vi "Line Main.vi"() -> ()   [LabVIEW 2020]
panel:
  in  "Send Image":bool
  in  "Image File Path":path
  out "Reply":string
  in  "Send Message":bool
  in  "Message":string
  in  "Token":string="zqz9UE9y1PFtpszUMYZdfwgDTmGI6nrZ7WZ0uJgGMP1"
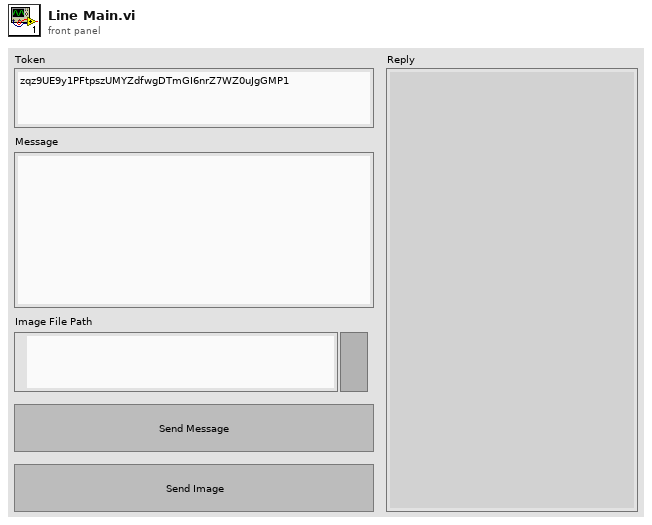
[diagram p1: front panel]
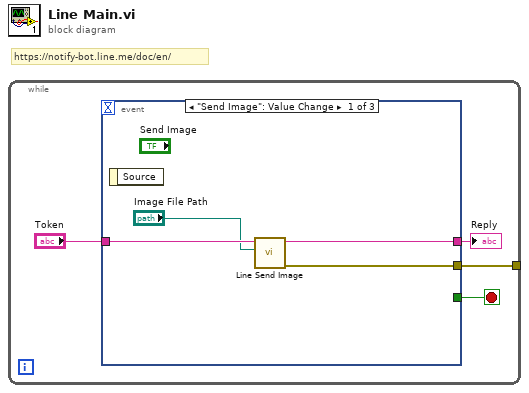
[diagram p0: block diagram]
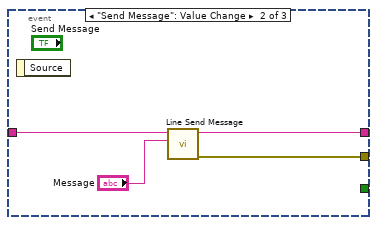
[diagram p2: hidden frame]
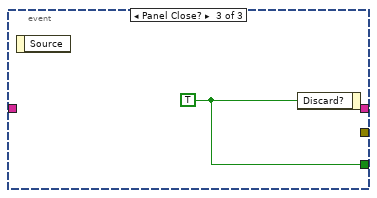
[diagram p3: hidden frame]
diagram:
  # "https://notify-bot.line.me/doc/en/"
  n1 = while {
    tunnel: [w2] -> _
    stop <- w3 stop-if-true
    n2 = event shown="[0] \"Send Image\": Value Change" {
      selector: _ -> [_ _ _]
      dyn-events: _ -> [_ _ _]
      timeout: _ -> [_ _ _]
      tunnel: "Token" -> [w8 w12 _]
      tunnel: [w7 w10 _] -> w2
      tunnel: [_ _ w13] -> w3
      tunnel: [w6 w9 _] -> w1
      event "Send Image": Value Change {
        n3 = event-data() -> ()  [unwired: 1 in, 1 out]
        n4 = call "Line Send Image.vi"("Image Path"="Image File Path", "Token"=w8) -> ("error out"=w7:errorcluster, "Reply"=w6:string)  [unwired: 8 in]
      }
      event "Send Message": Value Change {
        n5 = event-data() -> ()  [unwired: 1 in, 1 out]
        n6 = call "Line Send Message.vi"("Message"="Message", "Token"=w12) -> ("error out"=w10:errorcluster, "Reply"=w9:string)  [unwired: 8 in]
      }
      event Panel Close? {
        w13 = TRUE ("Discard?")
        n7 = event-data() -> ()  [unwired: 1 in, 1 out]
        n8 = event-data("Discard?"=w13) -> ()  [unwired: 1 in, 1 out]
      }
    }
    "Reply" <- w1
  }
